vi "get_ready_flag.vi"(8 "error in (no error)":errorcluster, 11 "GenericTrajectory in":refnum<class "GenericTrajectory.lvclass">) -> (0 "error out":errorcluster, 2 "ready for initialisation?":bool, 3 "GenericTrajectory out":refnum<class "GenericTrajectory.lvclass">)   [LabVIEW 2010, in "GenericTrajectory.lvclass"]
doc: "returns a flag indicating whether all defining parameters have been set and the Trajectory object is ready for initialisation"
uses:
  GenericTrajectory.lvclass
  GenericTrajectory.lvclass/GenericTrajectory.ctl
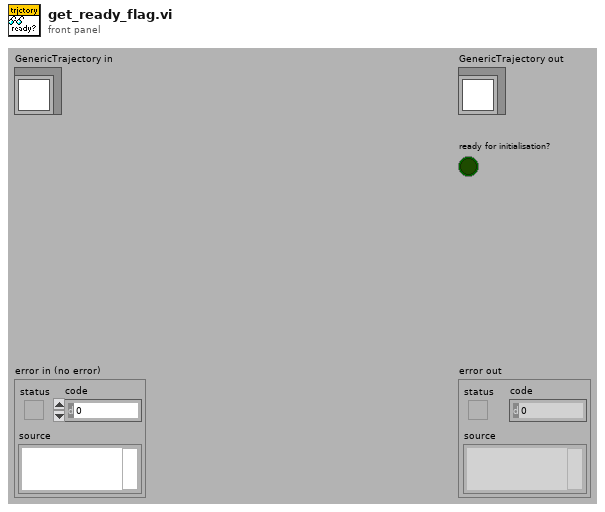
[diagram p1: front panel]
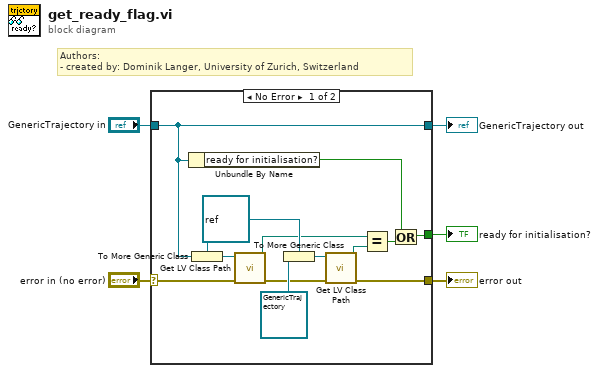
[diagram p0: block diagram]
diagram:
  # "Authors: \n- created by: Dominik Langer, University of Zurich, Switzerland"
  n1 = case shown="No Error" "error in (no error)" {
    selector: "error in (no error)" -> [w18 w19]
    tunnel: [w11 w19] -> w4
    tunnel: [w17 w20] -> w2
    tunnel: "GenericTrajectory in" -> [w17 w20]
    tunnel: [w6 _] -> w1
    frame No Error {
      w15 = refnum<class> refnum ("LabVIEW Object")
      n2 = Unbundle By Name(w17) -> ("ready for initialisation?"=w7:bool)
      n3 = To More Generic Class(target class=w15, reference=w17) -> (generic class reference=w16:refnum<class>)
      n4 = call <vilib>:"Get LV Class Path.vi"("error in (no error)"=w18, "object"=w16) -> ("error out"=w12:errorcluster, "class path"=w10:path)  [unwired: 8 in]
      n5 = To More Generic Class(target class=w15, reference=refnum<class "GenericTrajectory.lvclass"> refnum ("GenericTrajectory.lvclass")) -> (generic class reference=w13:refnum<class>)
      n6 = call <vilib>:"Get LV Class Path.vi"("error in (no error)"=w12, "object"=w13) -> ("error out"=w11:errorcluster, "class path"=w9:path)  [unwired: 8 in]
      n7 = Equal?(x=w10, y=w9) -> (x = y?=w8:bool)
      n8 = Or(x=w7, y=w8) -> (x .or. y?=w6:bool)
    }
    frame Error {
    }
  }
  "error out" <- w4
  "GenericTrajectory out" <- w2
  "ready for initialisation?" <- w1
